vi "load_sxp_file.vi"(6 "filename_in":string, 7 "button_load_s1p":bool, 8 "data_available_in":T1, 9 "freq_available in":bool, 10 "data_array_in":dbl[][](array[numeric]), 11 "freq_array_in":dbl[](array[numeric])) -> (0 "data_available_out":T1, 1 "freq_available out":bool, 2 "data_array_out":dbl[][](array[numeric]), 3 "freq_array_out":dbl[](array[numeric]), 4 "filename_out":string)   [LabVIEW 2025]
uses:
  <vilib>/Utility/error.llb/whitespace.ctl
  <vilib>/Utility/error.llb/Trim Whitespace One-Sided.vi
panel:
  out "Loaded *.sxp-File":string
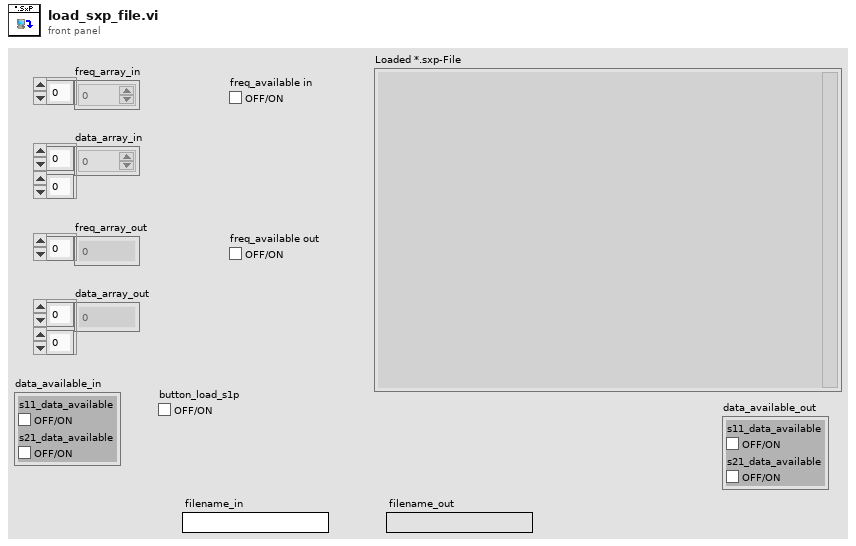
[diagram p1: front panel]
types:
  T1 = cluster{"s11_data_available":bool, "s21_data_available":bool}
  T2 = typedef "whitespace.ctl" = u16
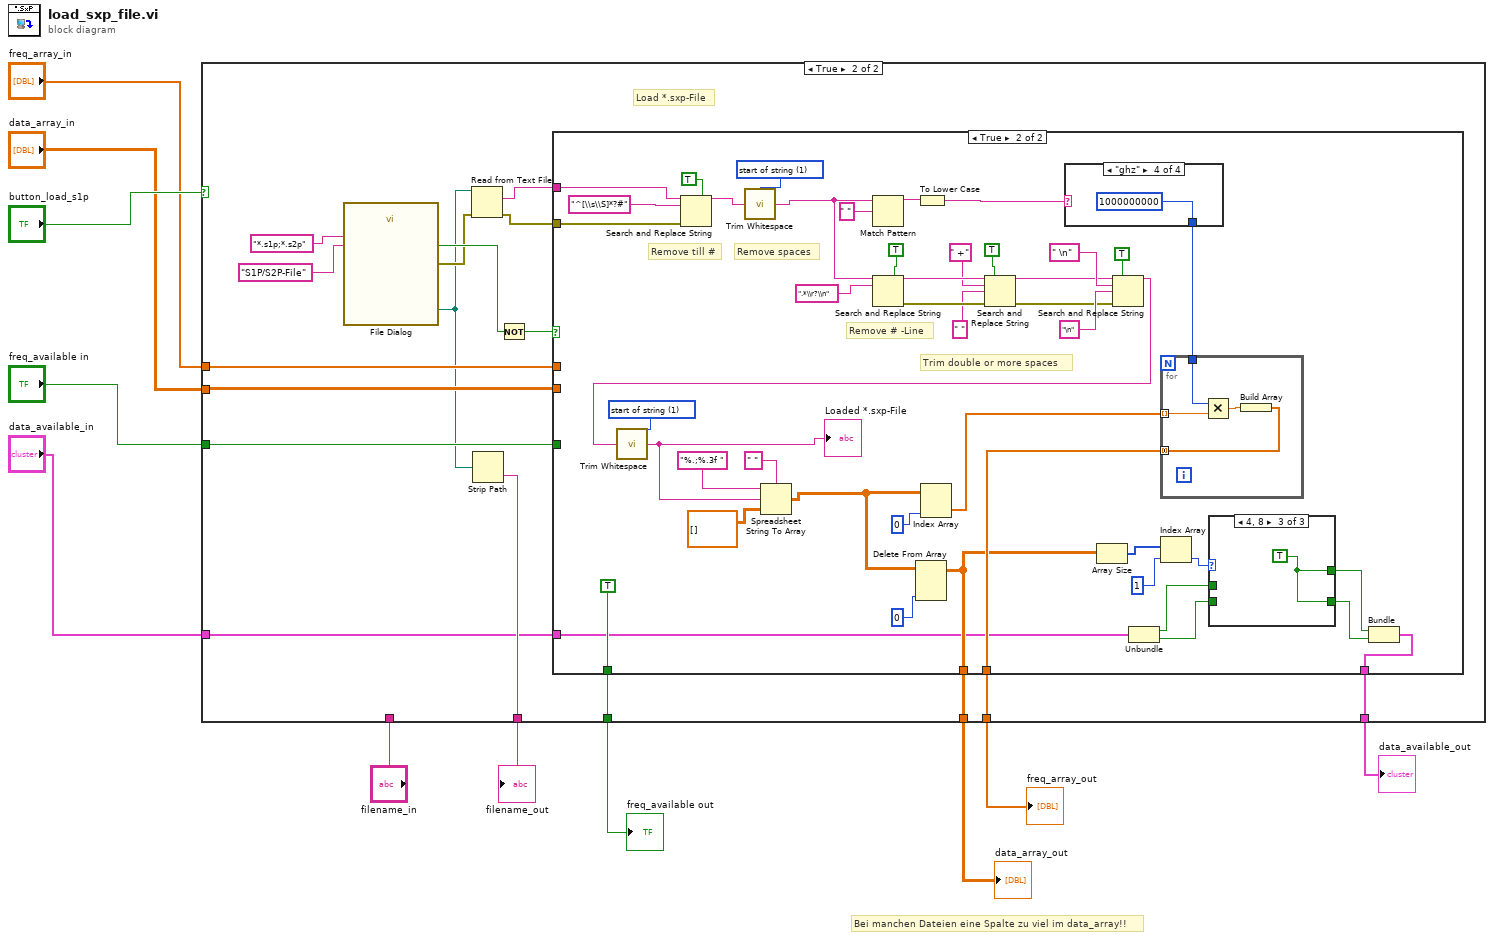
[diagram p0: block diagram]
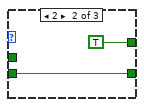
[diagram p5: hidden frame]
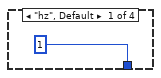
[diagram p6: hidden frame]
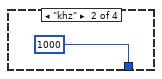
[diagram p7: hidden frame]
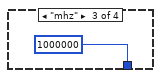
[diagram p8: hidden frame]
diagram:
  # "Bei manchen Dateien eine Spalte zu viel im data_array!!"
  n1 = case shown="True" "button_load_s1p" {
    tunnel: [w16 w33] -> w11
    tunnel: "freq_array_in" -> [w16 w21]
    tunnel: [w15 w32] -> w10
    tunnel: "data_array_in" -> [w15 w22]
    tunnel: [w14 w31] -> w8
    tunnel: "freq_available in" -> [w14 w23]
    tunnel: [w13 w19] -> w4
    tunnel: "filename_in" -> [w13 _]
    tunnel: "data_available_in" -> [w12 w18]
    tunnel: [w12 w17] -> w1
    frame False {
    }
    frame True {
      # "Load *.sxp-File"
      n2 = call "File Dialog"("pattern (all files)"="*.s1p;*.s2p" ("pattern label"), "pattern label"="S1P/S2P-File") -> ("selected path"=w20:path, "cancelled"=w28:bool, "error out"=w26:errorcluster)  [unwired: 10 in, 1 out]
      n3 = Read from Text File(file (use dialog)=w20, error in=w26) -> (text=w30:string, error out=w27:errorcluster)  [unwired: 2 in, 2 out]
      n4 = Strip Path(path=w20) -> (name=w19:string)  [unwired: 1 out]
      n5 = Not(x=w28) -> (.not. x?=w29:bool)
      n6 = case shown="True" w29 {
        tunnel: [w35 w54] -> w33
        tunnel: [w36 w53] -> w32
        tunnel: [w37 TRUE ("freq_available")] -> w31
        tunnel: w30 -> [_ w75]
        tunnel: w27 -> [_ w74]
        tunnel: w23 -> [w37 _]
        tunnel: w22 -> [w36 _]
        tunnel: w21 -> [w35 _]
        tunnel: w18 -> [w34 w49]
        tunnel: [w34 w42] -> w17
        frame False {
        }
        frame True {
          w67 = T2 1 items=["both", "start of string", "end of string"] ("location (both)")
          w71 = T2 1 items=["both", "start of string", "end of string"] ("location (both)")
          # "Remove # -Line"
          # "Trim double or more spaces"
          # "Remove spaces"
          # "Remove till #"
          n7 = Search and Replace String(multiline?=TRUE ("replace all? (F)"), input string=w75, search string="^[\\s\\S]*?#", error in=w74) -> (result string=w72:string)  [unwired: 4 in, 3 out]
          n8 = call <vilib>:"Trim Whitespace.vi"("string"=w72, "location (both)"=w71) -> ("trimmed string"=w66:string)
          n9 = Match Pattern(string=w66, regular expression=" ") -> (before substring=w69:string)  [unwired: 1 in, 3 out]
          n10 = Search and Replace String(multiline?=TRUE ("multiline? (F)"), input string=w66, search string=".*\\r?\\n") -> (result string=w61:string, error out=w60:errorcluster)  [unwired: 5 in, 2 out]
          n11 = To Lower Case(string=w69) -> (all lower case string=w68:string)
          n12 = Search and Replace String(replace all?=TRUE ("replace all? (F)"), input string=w61, search string=" +", replace string=" " ("replace string (\"\")"), error in=w60) -> (result string=w41:string, error out=w40:errorcluster)  [unwired: 3 in, 2 out]
          n13 = case shown="\"ghz\"" w68 {
            tunnel: [1 1000 1000000 1000000000] -> w56
            frame "hz", Default {
            }
            frame "khz" {
            }
            frame "mhz" {
            }
            frame "ghz" {
            }
          }
          n14 = Search and Replace String(replace all?=TRUE ("replace all? (F)"), input string=w41, search string=" \n", replace string="\n" ("replace string (\"\")"), error in=w40) -> (result string=w39:string)  [unwired: 3 in, 3 out]
          n15 = call <vilib>:"Trim Whitespace.vi"("string"=w39, "location (both)"=w67) -> ("trimmed string"=w62:string)
          "Loaded *.sxp-File" <- w62
          n16 = Spreadsheet String To Array(delimiter (Tab)=" " ("element"), format string="%.;%.3f ", spreadsheet string=w62, array type (2D Dbl)=dbl[][] []) -> (array=w63:dbl[][])
          n17 = Delete From Array(array=w63, index (col)=0) -> (array with subset deleted=w53:dbl[][])  [unwired: 2 in, 1 out]
          n18 = Index Array(array=w63, index (col)=0) -> (element=w55:dbl[])  [unwired: 1 in]
          n19 = Array Size(array=w53) -> (size(s)=w52:i32[])
          n20 = Unbundle(w49) -> ("s11_data_available"=w45:bool, "s21_data_available"=w47:bool)
          n21 = for {
            tunnel: w56 -> [w91]
            tunnel: w55 -> [w90] mode=indexing
            tunnel: [w88] -> w54 mode=concatenating
            n22 = Multiply(x=w91, y=w90) -> (x*y=w89:dbl)
            n23 = Build Array(w89) -> (w88:dbl[])
          }
          n24 = Index Array(array=w52, index=1) -> (element=w50:i32)
          n25 = case shown="4, 8" w50 {
            tunnel: [w83 w86 w87] -> w48
            tunnel: w47 -> [w83 w86 _]
            tunnel: [w84 TRUE w87] -> w46
            tunnel: w45 -> [w84 _ _]
            frame 0, Default {
            }
            frame 2 {
            }
            frame 4, 8 {
              w87 = TRUE
            }
          }
          n26 = Bundle("s11_data_available"=w46, "s21_data_available"=w48) -> (w42:T1)  [unwired: 1 in]
        }
      }
    }
  }
  "freq_array_out" <- w11
  "data_array_out" <- w10
  "freq_available out" <- w8
  "filename_out" <- w4
  "data_available_out" <- w1
